vi "Send Command.vi"(8 "error in (no error)":errorcluster, 10 "operation":u32 format="%.0x", 11 "device index":i8) -> (0 "error out":errorcluster, 2 "Result":u32, 3 "device index out":i8)   [LabVIEW 2015, in "HD44780 FPGA.lvlib"]
uses:
  <vilib>/EmbeddedDisplay/Hitachi HD44780/FPGA/HD44780 FPGA.lvlib
  <vilib>/EmbeddedDisplay/Hitachi HD44780/FPGA/Internal/LCD Command.vi
  <vilib>/EmbeddedDisplay/Hitachi HD44780/Common/HD44780 Common.lvlib
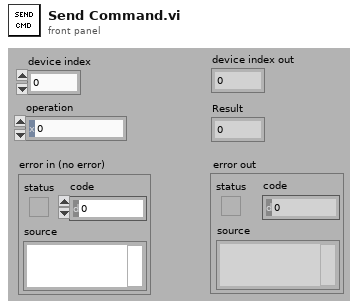
[diagram p1: front panel]
types:
  T1 = cluster{"device index (-1)":i8, "operation (0)":u32}
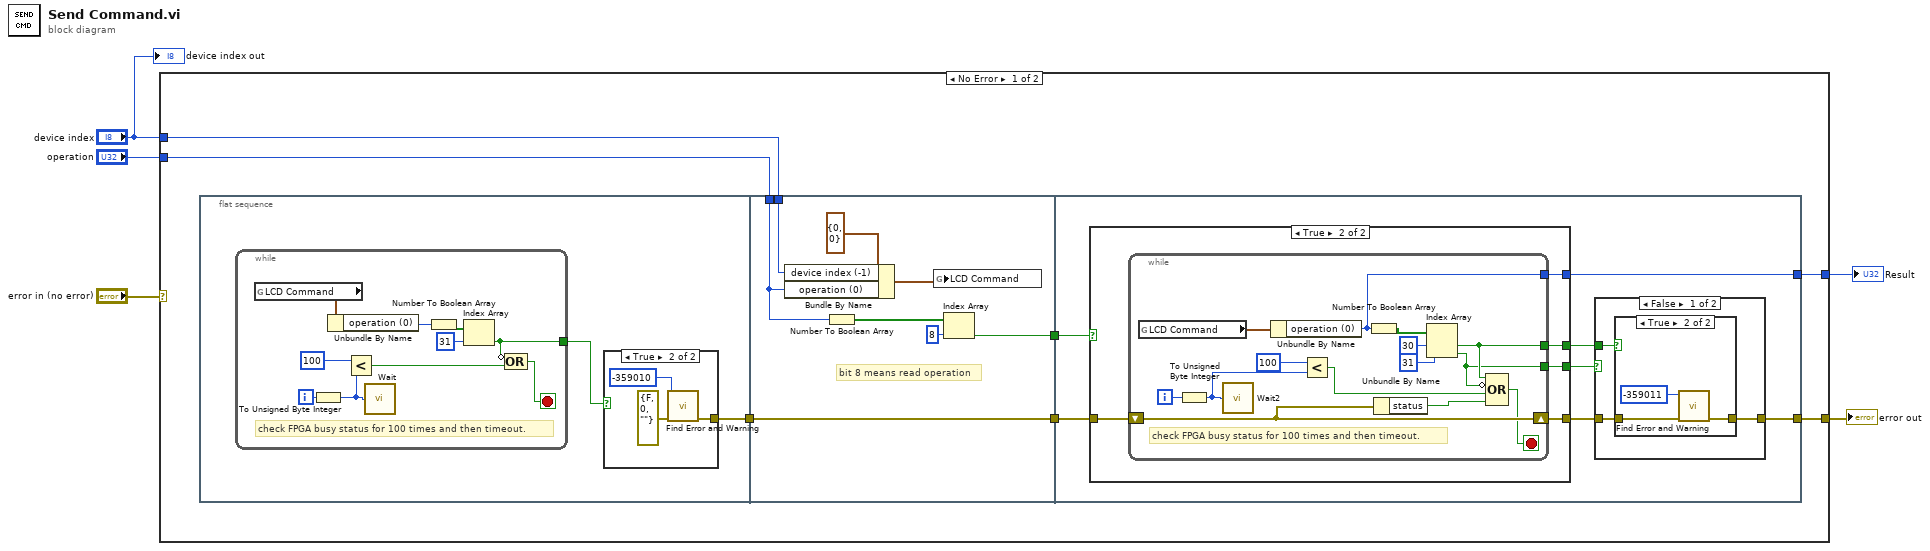
[diagram p0: block diagram]
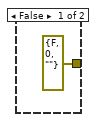
[diagram p2: hidden frame]
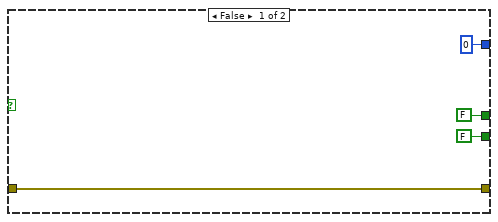
[diagram p3: hidden frame]
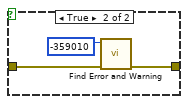
[diagram p5: hidden frame]
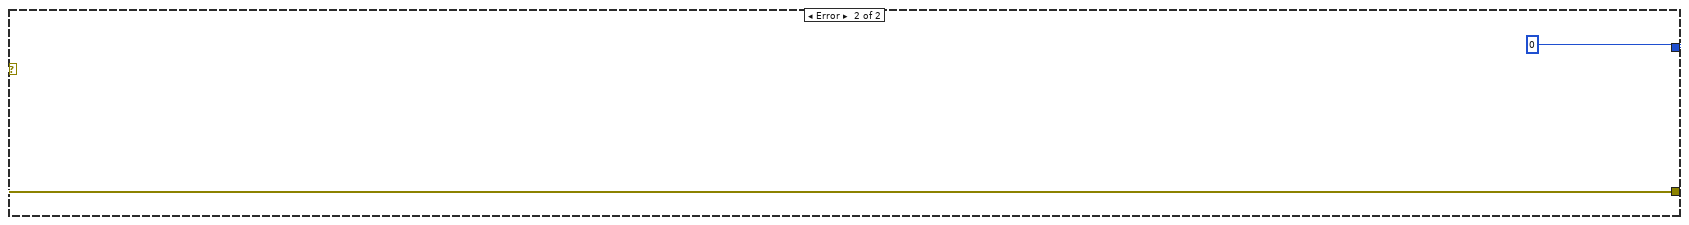
[diagram p6: hidden frame]
diagram:
  n1 = case shown="No Error" "error in (no error)" {
    selector: "error in (no error)" -> [_ w78]
    tunnel: [w12 u32 0 ("operation")] -> w5
    tunnel: "device index" -> [w8 _]
    tunnel: "operation" -> [w7 _]
    tunnel: [w11 w78] -> w1
    frame No Error {
      n2 = flat-sequence {
        tunnel: [w14] -> w10
        tunnel: w10 -> [w36]
        tunnel: [w36] -> w9
        tunnel: w8 -> [w31]
        tunnel: w7 -> [w29]
        tunnel: [w30] -> w6
        tunnel: w9 -> [w39]
        tunnel: [w40] -> w11
        tunnel: [w38] -> w12
        tunnel: w6 -> [w37]
        frame #0 {
          n3 = while {
            tunnel: [w17] -> w13
            i -> [w20]
            stop <- w15 stop-if-true
            # "check FPGA busy status for 100 times and then timeout."
            n4 = global read "LCD Command.vi" "LCD Command"() -> (w21:T1)
            n5 = To Unsigned Byte Integer(number=w20) -> (unsigned 8bit integer=w18:u8)
            n6 = Unbundle By Name(w21) -> ("operation (0)"=w24:u32)
            n7 = Less?(x=u8 100, y=w18) -> (x < y?=w16:bool)
            n8 = call "Wait"("Count(mSec)"=w18) -> ()  [unwired: 1 out]
            n9 = Number To Boolean Array(number=w24) -> (Boolean array=w23:bool[])
            n10 = Index Array(array=w23, index=31) -> (element=w17:bool)
            n11 = Compound Arithmetic op=OR(invert w17, w16) -> (w15:bool)
          }
          n12 = case shown="True" w13 {
            tunnel: [errorcluster {"status"=FALSE, "code"=0, "source"=""} ("error out") w26] -> w14
            frame False {
            }
            frame True {
              n13 = call <vilib>:"Find Error and Warning.vi"("error in (no error)"=errorcluster {"status"=FALSE, "code"=0, "source"=""}, "error code"=-359010) -> ("error out"=w26:errorcluster)  [unwired: 9 in]
            }
          }
        }
        frame #1 {
          # "bit 8 means read operation"
          n14 = Bundle By Name(cluster=T1 {"device index (-1)"=0, "operation (0)"=0} ("LCD Command"), "device index (-1)"=w31, "operation (0)"=w29) -> (w33:T1)
          n15 = Number To Boolean Array(number=w29) -> (Boolean array=w34:bool[])
          n16 = global write "LCD Command.vi" "LCD Command"(w33) -> ()
          n17 = Index Array(array=w34, index=8) -> (element=w30:bool)
        }
        frame #2 {
          n18 = case shown="True" w37 {
            tunnel: w39 -> [w45 w52]
            tunnel: [FALSE w51] -> w43
            tunnel: [FALSE w50] -> w42
            tunnel: [w45 w49] -> w41
            tunnel: [u32 0 ("operation (0)") w48] -> w38
            frame False {
            }
            frame True {
              n19 = while {
                shift-right: [w61] -> w49
                shift-left: w52 -> [w61]
                tunnel: [w60] -> w51
                tunnel: [w59] -> w50
                tunnel: [w53] -> w48
                i -> [w64]
                stop <- w56 stop-if-true
                # "check FPGA busy status for 100 times and then timeout."
                n20 = global read "LCD Command.vi" "LCD Command"() -> (w65:T1)
                n21 = To Unsigned Byte Integer(number=w64) -> (unsigned 8bit integer=w57:u8)
                n22 = call "Wait2"("Count(mSec)"=w57) -> ()  [unwired: 1 out]
                n23 = Unbundle By Name(w65) -> ("operation (0)"=w53:u32)
                n24 = Less?(x=u8 100, y=w57) -> (x < y?=w54:bool)
                n25 = Number To Boolean Array(number=w53) -> (Boolean array=w66:bool[])
                n26 = Unbundle By Name(w61) -> ("status"=w55:bool)
                n27 = Index Array(array=w66, index #1=30 ("index"), index #2=31 ("index")) -> (element #1=w60:bool, element #2=w59:bool)
                n28 = Compound Arithmetic op=OR(w60, invert w59, w54, w55) -> (w56:bool)
              }
            }
          }
          n29 = case shown="False" w42 {
            tunnel: [w68 w75] -> w40
            tunnel: w41 -> [w69 w76]
            tunnel: w43 -> [w67 _]
            frame False {
              n30 = case shown="True" w67 {
                tunnel: w69 -> [w70 w72]
                tunnel: [w70 w71] -> w68
                frame False {
                }
                frame True {
                  n31 = call <vilib>:"Find Error and Warning.vi"("error in (no error)"=w72, "error code"=-359011) -> ("error out"=w71:errorcluster)  [unwired: 9 in]
                }
              }
            }
            frame True {
              n32 = call <vilib>:"Find Error and Warning.vi"("error in (no error)"=w76, "error code"=-359010) -> ("error out"=w75:errorcluster)  [unwired: 9 in]
            }
          }
        }
      }
    }
    frame Error {
    }
  }
  "Result" <- w5
  "error out" <- w1
  "device index out" <- "device index"
